vi "User Events - Register Events.vi"(8 "error in":errorcluster) -> (0 "error out":errorcluster, 3 "Event Registration Out":refnum<event-registration>)   [LabVIEW 2024, in "User Events.lvlib"]
uses:
  User Events.lvlib
  General Type Defs/User Events Cluster.ctl
  General Type Defs/FGV States.ctl
  General Type Defs/General Type Definitions.lvlib
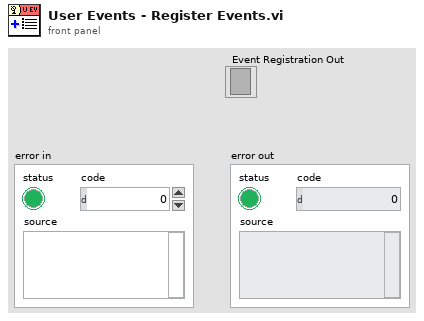
[diagram p1: front panel]
types:
  T1 = typedef "General Type Definitions.lvlib/FGV States.ctl" = enum16{"Create", "Get", "Destroy"}
  T2 = typedef "General Type Definitions.lvlib/User Events Cluster.ctl" = cluster{"STOP":refnum<user-event>, "Timeout":refnum<user-event>, "Error":refnum<user-event>}
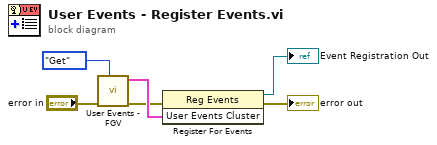
[diagram p0: block diagram]
diagram:
  n1 = call "User Events - FGV.vi"("FGV States"=FGV_States."Get", "error in"="error in") -> ("error out"=w2:errorcluster, "User Events Cluster"=w3:T2)  [unwired: 8 in]
  n2 = register-events(error in=w2, w3) -> (reference out=→"Event Registration Out":refnum<event-registration>, error out=→"error out":errorcluster)  [unwired: 1 in]
